vi "Enforce Robot Rules.vi"(9 "Disable":bool, 10 "New Points":cluster{"x":dbl, "y":dbl, "th":dbl}[](array[cluster]), 11 "Original Points":cluster{"x":dbl, "y":dbl, "th":dbl}[](array[cluster])) -> (3 "Points out":cluster{"x":dbl, "y":dbl, "th":dbl}[](array[cluster]))   [LabVIEW 2018]
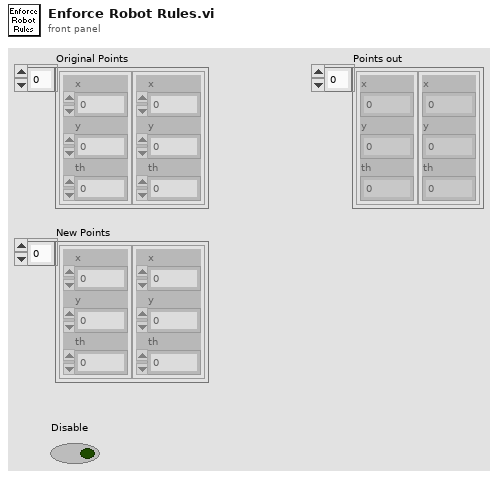
[diagram p1: front panel]
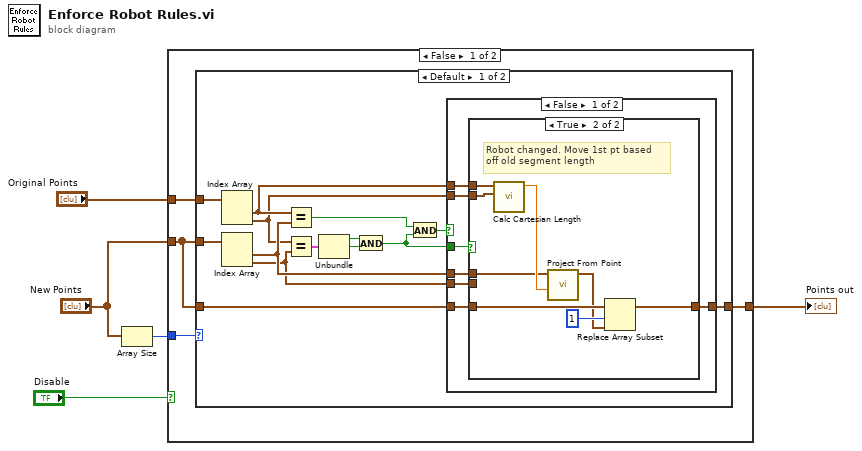
[diagram p0: block diagram]
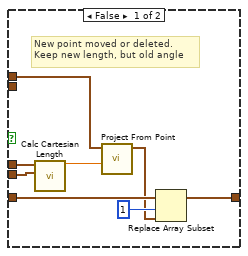
[diagram p2: hidden frame]
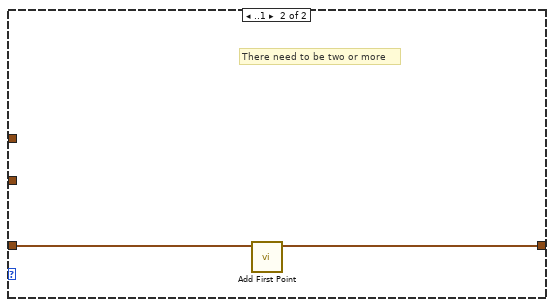
[diagram p4: hidden frame]
diagram:
  n1 = Array Size(array="New Points") -> (size(s)=w4:i32)
  n2 = case shown="False" "Disable" {
    tunnel: "Original Points" -> [w9 _]
    tunnel: w4 -> [w8 _]
    tunnel: [w7 w50] -> w3
    tunnel: "New Points" -> [w6 w50]
    frame False {
      n3 = case shown="Default" w8 {
        tunnel: w9 -> [w23 _]
        tunnel: w6 -> [w22 _]
        tunnel: [w20 w49] -> w7
        tunnel: w6 -> [w19 w48]
        frame Default {
          n4 = Index Array(array=w23) -> (element #1=w17:cluster{"x":dbl, "y":dbl, "th":dbl}, element #2=w14:cluster{"x":dbl, "y":dbl, "th":dbl})  [unwired: 2 in]
          n5 = Index Array(array=w22) -> (element #1=w16:cluster{"x":dbl, "y":dbl, "th":dbl}, element #2=w15:cluster{"x":dbl, "y":dbl, "th":dbl})  [unwired: 2 in]
          n6 = Equal?(x=w17, y=w16) -> (x = y?=w18:bool)
          n7 = Equal?(x=w14, y=w15) -> (x = y?=w13:cluster{"x":bool, "y":bool, "th":bool})
          n8 = Unbundle(w13) -> ("x"=w12:bool, "y"=w11:bool)  [unwired: 1 out]
          n9 = And(x=w12, y=w11) -> (x .and. y?=w10:bool)
          n10 = And(x=w18, y=w10) -> (x .and. y?=w21:bool)
          n11 = case shown="False" w21 {
            tunnel: [w26 w47] -> w20
            tunnel: w19 -> [w24 w47]
            tunnel: w10 -> [w28 _]
            tunnel: w17 -> [w30 _]
            tunnel: w14 -> [w29 _]
            tunnel: w16 -> [w27 _]
            tunnel: w15 -> [w25 _]
            frame False {
              n12 = case shown="True" w28 {
                tunnel: w30 -> [w33 w46]
                tunnel: w29 -> [_ w45]
                tunnel: w27 -> [w38 w40]
                tunnel: [w34 w43] -> w26
                tunnel: w25 -> [w37 _]
                tunnel: w24 -> [w35 w44]
                frame False {
                  # "New point moved or deleted.\nKeep new length, but old angle"
                  n13 = call "Calc Cartesian Length.vi"("Point 2"=w37, "Point 1"=w38) -> ("Length (f)"=w32:dbl)  [unwired: 8 in, 1 out]
                  n14 = call "Project From Point.vi"("distance"=w32, "Point In"=w33) -> ("Point Out"=w31:cluster{"x":dbl, "y":dbl, "th":dbl})  [unwired: 9 in]
                  n15 = Replace Array Subset(array=w35, new element=w31, index=1) -> (w34:cluster{"x":dbl, "y":dbl, "th":dbl}[])
                }
                frame True {
                  # "Robot changed. Move 1st pt based\noff old segment length"
                  n16 = call "Calc Cartesian Length.vi"("Point 2"=w45, "Point 1"=w46) -> ("Length (f)"=w41:dbl)  [unwired: 8 in, 1 out]
                  n17 = call "Project From Point.vi"("distance"=w41, "Point In"=w40) -> ("Point Out"=w39:cluster{"x":dbl, "y":dbl, "th":dbl})  [unwired: 9 in]
                  n18 = Replace Array Subset(array=w44, new element=w39, index=1) -> (w43:cluster{"x":dbl, "y":dbl, "th":dbl}[])
                }
              }
            }
            frame True {
              # "First two elements didn't\nchange. assume they are\ngood"
            }
          }
        }
        frame ..1 {
          # "There need to be two or more"
          n19 = call "Add First Point.vi"("Initial Points"=w48) -> ("Points"=w49:cluster{"x":dbl, "y":dbl, "th":dbl}[])  [unwired: 10 in]
        }
      }
    }
    frame True {
    }
  }
  "Points out" <- w3
